vi "Post Step Temperature Engine Stop.vi"() -> (0 "error out":errorcluster, 3 "Report Text":string)   [LabVIEW 2023, in "LTT_TeststandSteptypes.lvlib"]
uses:
  LTT_TeststandSteptypes.lvlib
panel:
  out "Report Text":string
  in  "Sequence Context In":refnum<k7>
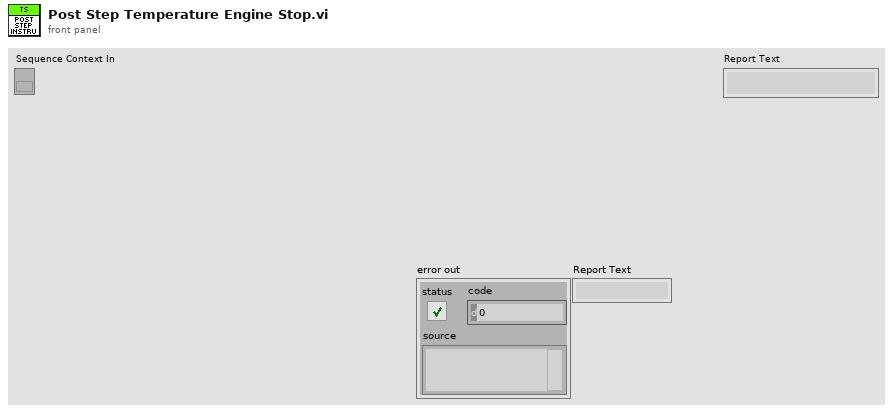
[diagram p1: front panel]
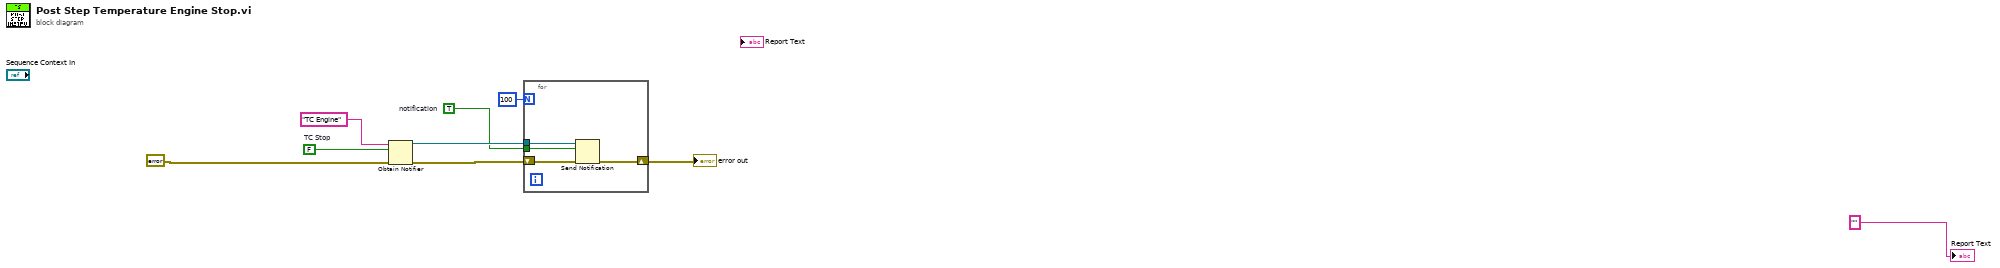
[diagram p0: block diagram]
diagram:
  w2 = TRUE  # notification
  w5 = FALSE  # TC Stop
  n1 = Obtain Notifier(name (unnamed)="TC Engine", notification data type=w5, error in (no error)=errorcluster {"status"=FALSE, "code"=0, "source"=""}) -> (notifier out=w4:refnum<notifier>, error out=w3:errorcluster)  [unwired: 1 in, 1 out]
  n2 = for {
    N: 100 -> [_]
    tunnel: w4 -> [w13]
    tunnel: w2 -> [w11]
    shift-right: [w10] -> w8
    shift-left: w3 -> [w12]
    n3 = Send Notification(notification=w11, notifier=w13, error in (no error)=w12) -> (error out=w10:errorcluster)  [unwired: 1 out]
  }
  "error out" <- w8
  "Report Text" <- "" ("delimiter (Tab)")
